vi "Configure Standard Waveform Frequency.vi"(0 "VISA resource name":refnum<visa-resource-name>, 1 "Frequency (1000 Hz)":dbl=1000.0, 5 "Channel (0: Channel 1)":u16(ring) items=["Channel 1", "Channel 2"], 7 "Waveform Function (0: Sine)":u16(ring) items=["Sine", "Square", "Pulse", "Ramp", "Noise", "DC", "Sin(x)/x", "Gaussian", "Lorentz", "Exponential Rise", "Exponential Decay", "Haversine"], 11 "error in (no error)":errorcluster) -> (4 "VISA resource name out":refnum<visa-resource-name>, 15 "error out":errorcluster)   [LabVIEW 2020, in "AWG.lvlib" / "Tektronix AFG 3000 Series.lvlib"]
doc: "Selects the waveform shape, frequency, amplitude, offset, and phase for a standard waveform."
uses:
  Tektronix AFG 3000 Series.lvlib
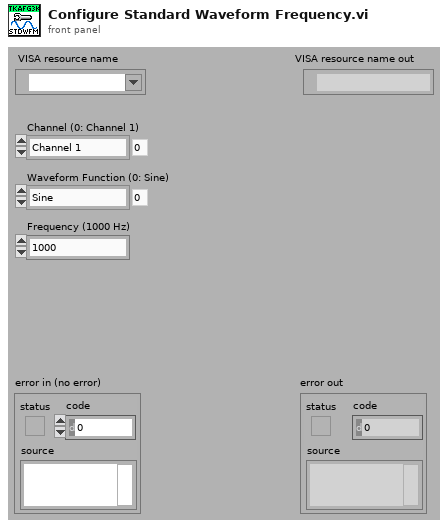
[diagram p1: front panel]
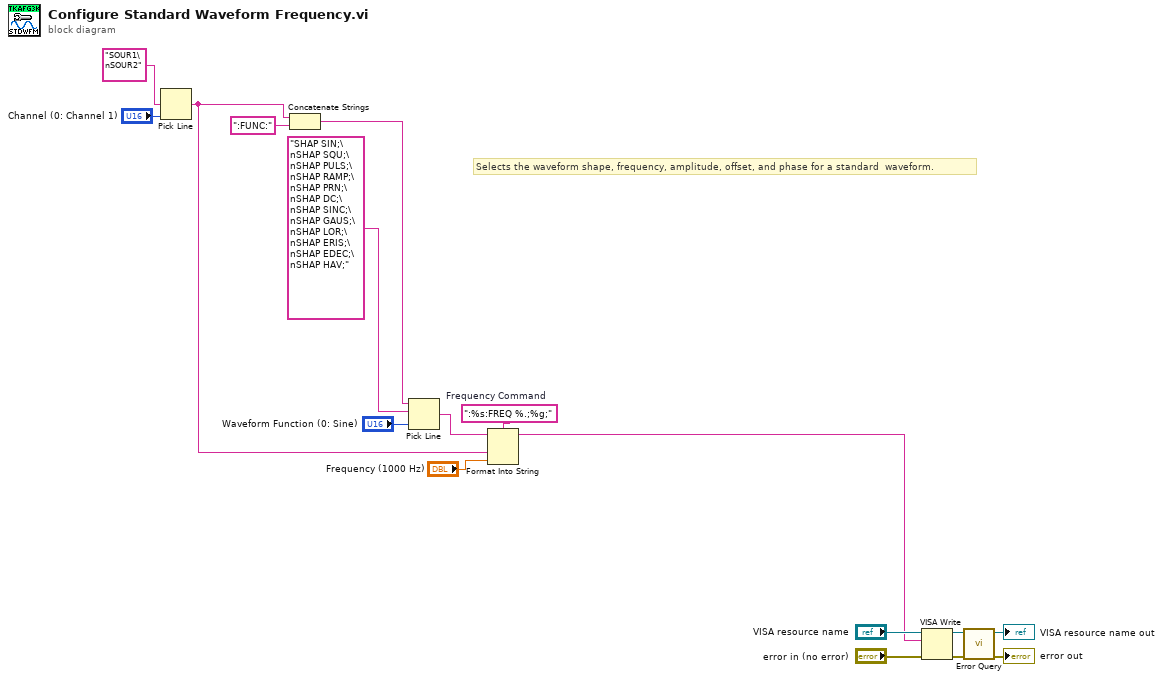
[diagram p0: block diagram]
diagram:
  w9 = ":%s:FREQ %.;%g;"  # Frequency Command
  # "Selects the waveform shape, frequency, amplitude, offset, and phase for a standard  waveform."
  n1 = Pick Line(multi-line string="SOUR1\nSOUR2" ("string (\"\")"), line index="Channel (0: Channel 1)") -> (output string=w3:string)  [unwired: 1 in]
  n2 = Concatenate Strings(w3, ":FUNC:" ("string")) -> (w5:string)
  n3 = Pick Line(string ("")=w5, multi-line string="SHAP SIN;\nSHAP SQU;\nSHAP PULS;\nSHAP RAMP;\nSHAP PRN;\nSHAP DC;\nSHAP SINC;\nSHAP GAUS;\nSHAP LOR;\nSHAP ERIS;\nSHAP EDEC;\nSHAP HAV;" ("Function Command"), line index="Waveform Function (0: Sine)") -> (output string=w1:string)
  n4 = Format Into String(format string=w9, initial string=w1, w3, "Frequency (1000 Hz)") -> (resulting string=w2:string)  [unwired: 1 in, 1 out]
  n5 = VISA Write(VISA resource name="VISA resource name", write buffer=w2, error in (no error)="error in (no error)") -> (VISA resource name out=w13:refnum<visa-resource-name>, error out=w12:errorcluster)  [unwired: 1 out]
  n6 = call "Error Query.vi"("error in (no error)"=w12, "VISA resource name"=w13) -> ("error out"=→"error out":errorcluster, "VISA resource name out"=→"VISA resource name out":refnum<visa-resource-name>)  [unwired: 6 in, 2 out]
